vi "Read Control Tags.vi"(10 "Paramaters  allocation in":T2, 11 "Sequencer Module runtime in":refnum<class "Sequencer Module runtime.lvclass">) -> (1 "Sequence Control":T1, 2 "Parameters allocation out":T2, 3 "Sequencer Module runtime out":refnum<class "Sequencer Module runtime.lvclass">)   [LabVIEW 2018, in "Sequencer Module runtime.lvclass"]
uses:
  Sequencer Module runtime.lvclass
  <vilib>/NI/Tag Bus/table/data table.ctl
  Sequencer Control.ctl
  Sequencer Module runtime.lvclass/Sequencer Module runtime.ctl
  <vilib>/NI/Tag Bus/table/data polymorphs/read one/read Boolean.vi
  <vilib>/NI/Tag Bus/table/data polymorphs/read one/read I32.vi
  <vilib>/NI/Tag Bus/table/data table.lvlib
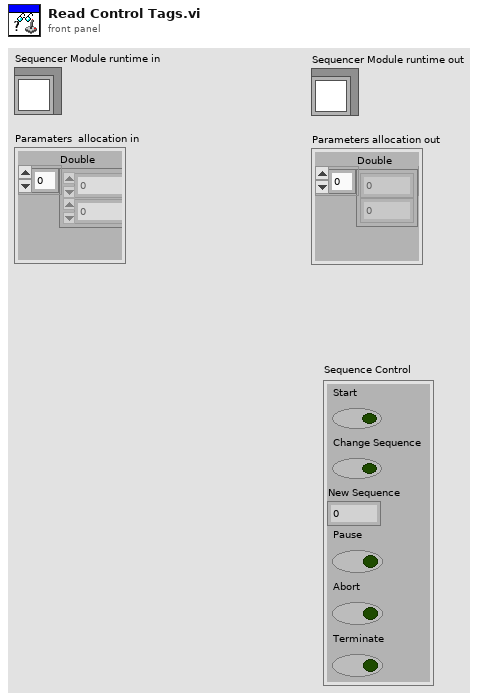
[diagram p1: front panel]
types:
  T1 = typedef "Sequencer Module runtime.lvclass/Sequencer Control.ctl" = cluster{"Start":bool, "Change Sequence":bool, "New Sequence":i32, "Pause":bool, "Abort":bool, "Terminate":bool}
  T2 = typedef "tag bus.lvlib/data table.lvlib/data table.ctl" = cluster{"Double":dbl[], "Single":sgl[], "I64":i64[], "I32":i32[], "I16":i16[], "I8":i8[], "U64":u64[], "U32":u32[], "U16":u16[], "U8":u8[], "Boolean":bool[], "String":string[], "Array of Double":cluster{"DBL Array":dbl[]}[], "Array of Single":cluster{"SGL Array":sgl[]}[], "Array of I64":cluster{"I64 Array":i64[]}[], "Array of I32":cluster{"I32 Array":i32[]}[], "Array of I16":cluster{"I16 Array":i16[]}[], "Array of I8":cluster{"I8 Array":i8[]}[], "Array of U64":cluster{"U64 Array":u64[]}[], "Array of U32":cluster{"U32 Array":u32[]}[], "Array of U16":cluster{"U16 Array":u16[]}[], "Array of U8":cluster{"U8 Array":u8[]}[], "Array of Boolean":cluster{"Boolean Array":bool[]}[], "Array of String":cluster{"String Array":string[]}[]}
  T3 = typedef "Sequencer Module runtime.lvclass/Sequencer Control Index.ctl" = cluster{"Start":i32, "Change Sequence":i32, "New Sequence":i32, "Pause":i32}
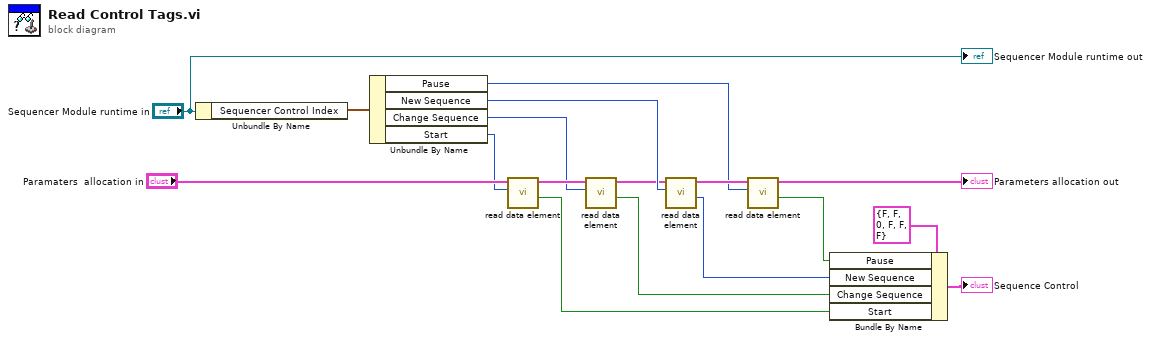
[diagram p0: block diagram]
diagram:
  n1 = Unbundle By Name("Sequencer Module runtime in") -> ("Sequencer Control Index"=w16:T3)
  n2 = Unbundle By Name(w16) -> ("Pause"=w3:i32, "New Sequence"=w15:i32, "Change Sequence"=w2:i32, "Start"=w4:i32)
  n3 = call-poly <vilib>:"read data element.vi"("index"=w4, "data table in"="Paramaters  allocation in") -> ("value"=w5:bool, "data table out"=w13:T2)  [unwired: 8 in]
  n4 = call-poly <vilib>:"read data element.vi"("index"=w2, "data table in"=w13) -> ("value"=w10:bool, "data table out"=w12:T2)  [unwired: 8 in]
  n5 = call-poly <vilib>:"read data element.vi"("index"=w15, "data table in"=w12) -> ("value"=w6:i32, "data table out"=w11:T2)  [unwired: 8 in]
  n6 = call-poly <vilib>:"read data element.vi"("index"=w3, "data table in"=w11) -> ("value"=w1:bool, "data table out"=→"Parameters allocation out":T2)  [unwired: 8 in]
  n7 = Bundle By Name(cluster=T1 {"Start"=FALSE, "Change Sequence"=FALSE, "New Sequence"=0, "Pause"=FALSE, "Abort"=FALSE, "Terminate"=FALSE} ("Sequence Control"), "Pause"=w1, "New Sequence"=w6, "Change Sequence"=w10, "Start"=w5) -> (→"Sequence Control":T1)
  "Sequencer Module runtime out" <- "Sequencer Module runtime in"
